vi "SetVoltage.vi"(8 "error in (no error)":errorcluster, 11 "B&K_Precision in":refnum<class "B&K_Precision.lvclass">) -> (0 "error out":errorcluster, 3 "B&K_Precision out":refnum<class "B&K_Precision.lvclass">)   [LabVIEW 2024, in "B&K_Precision.lvclass"]
uses:
  B&K_Precision.lvclass
  B&K_Precision.lvclass/B&K_Precision.ctl
  MainClass/PowerSupply.lvclass
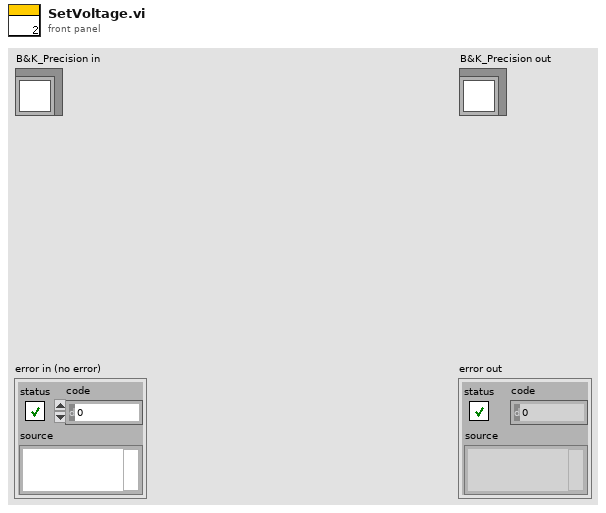
[diagram p1: front panel]
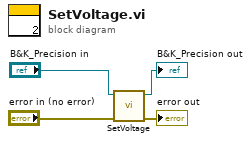
[diagram p0: block diagram]
diagram:
  n1 = call-parent "SetVoltage.vi"("error in (no error)"="error in (no error)", "PowerSupply in"="B&K_Precision in") -> ("error out"=→"error out":errorcluster, "PowerSupply out"=→"B&K_Precision out":refnum<class "B&K_Precision.lvclass">)  [unwired: 8 in]
